vi "VerasonicsTimeStamp.vi"(11 "Array":i16[][](array[numeric])) -> (3 "Numeric":u32)   [LabVIEW 2022 SP3]
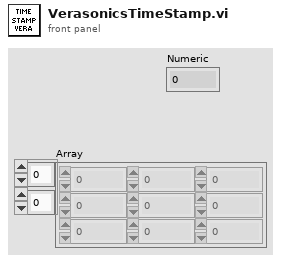
[diagram p1: front panel]
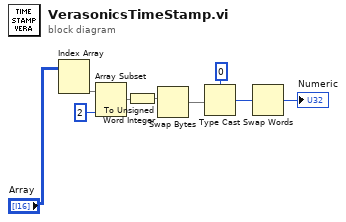
[diagram p0: block diagram]
diagram:
  n1 = Index Array(array="Array") -> (element=w9:i16[])  [unwired: 2 in]
  n2 = Array Subset(array=w9, length=2) -> (w4:i16[])  [unwired: 1 in]
  n3 = To Unsigned Word Integer(number=w4) -> (unsigned 16bit integer=w5:u16[])
  n4 = Swap Bytes(anything=w5) -> (byte swapped=w6:u16[])
  n5 = Type Cast(type=u32 0, x=w6) -> (*(type *) &x=w7:u32)
  n6 = Swap Words(1:w7) -> (0:→"Numeric":u32)
